vi "car proceed.vi"(0 "location in":T1, 1 "old buffer":T2, 2 "velocity in":cluster{"x":dbl, "y":dbl}, 3 "sensor reading":T3, 4 "Backward?":bool, 5 "refresh rate":i32) -> (6 "location out":T1, 8 "new buffer":T2, 9 "realdir":dbl, 10 "velocity out":cluster{"x":dbl, "y":dbl})   [LabVIEW 2020]
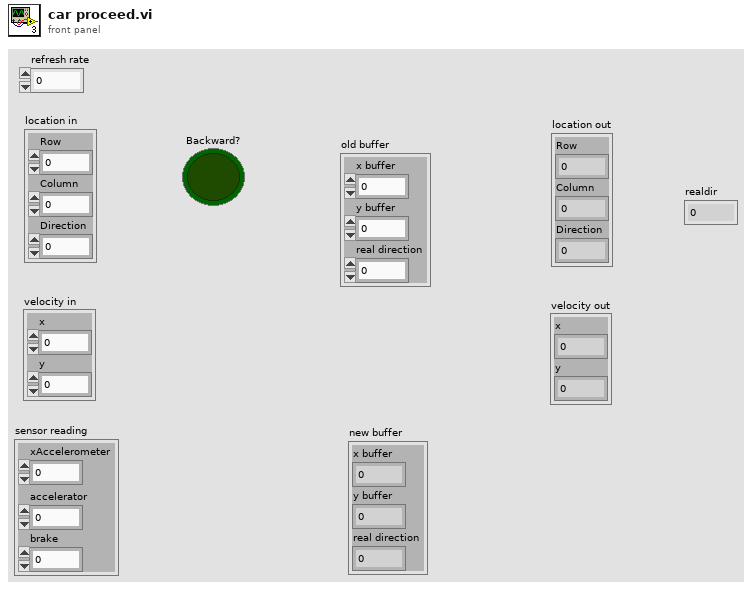
[diagram p1: front panel]
types:
  T1 = cluster{"Row":i32, "Column":i32, "Direction":i32}
  T2 = cluster{"x buffer":dbl, "y buffer":dbl, "real direction":dbl}
  T3 = cluster{"xAccelerometer":dbl, "accelerator":dbl, "brake":dbl}
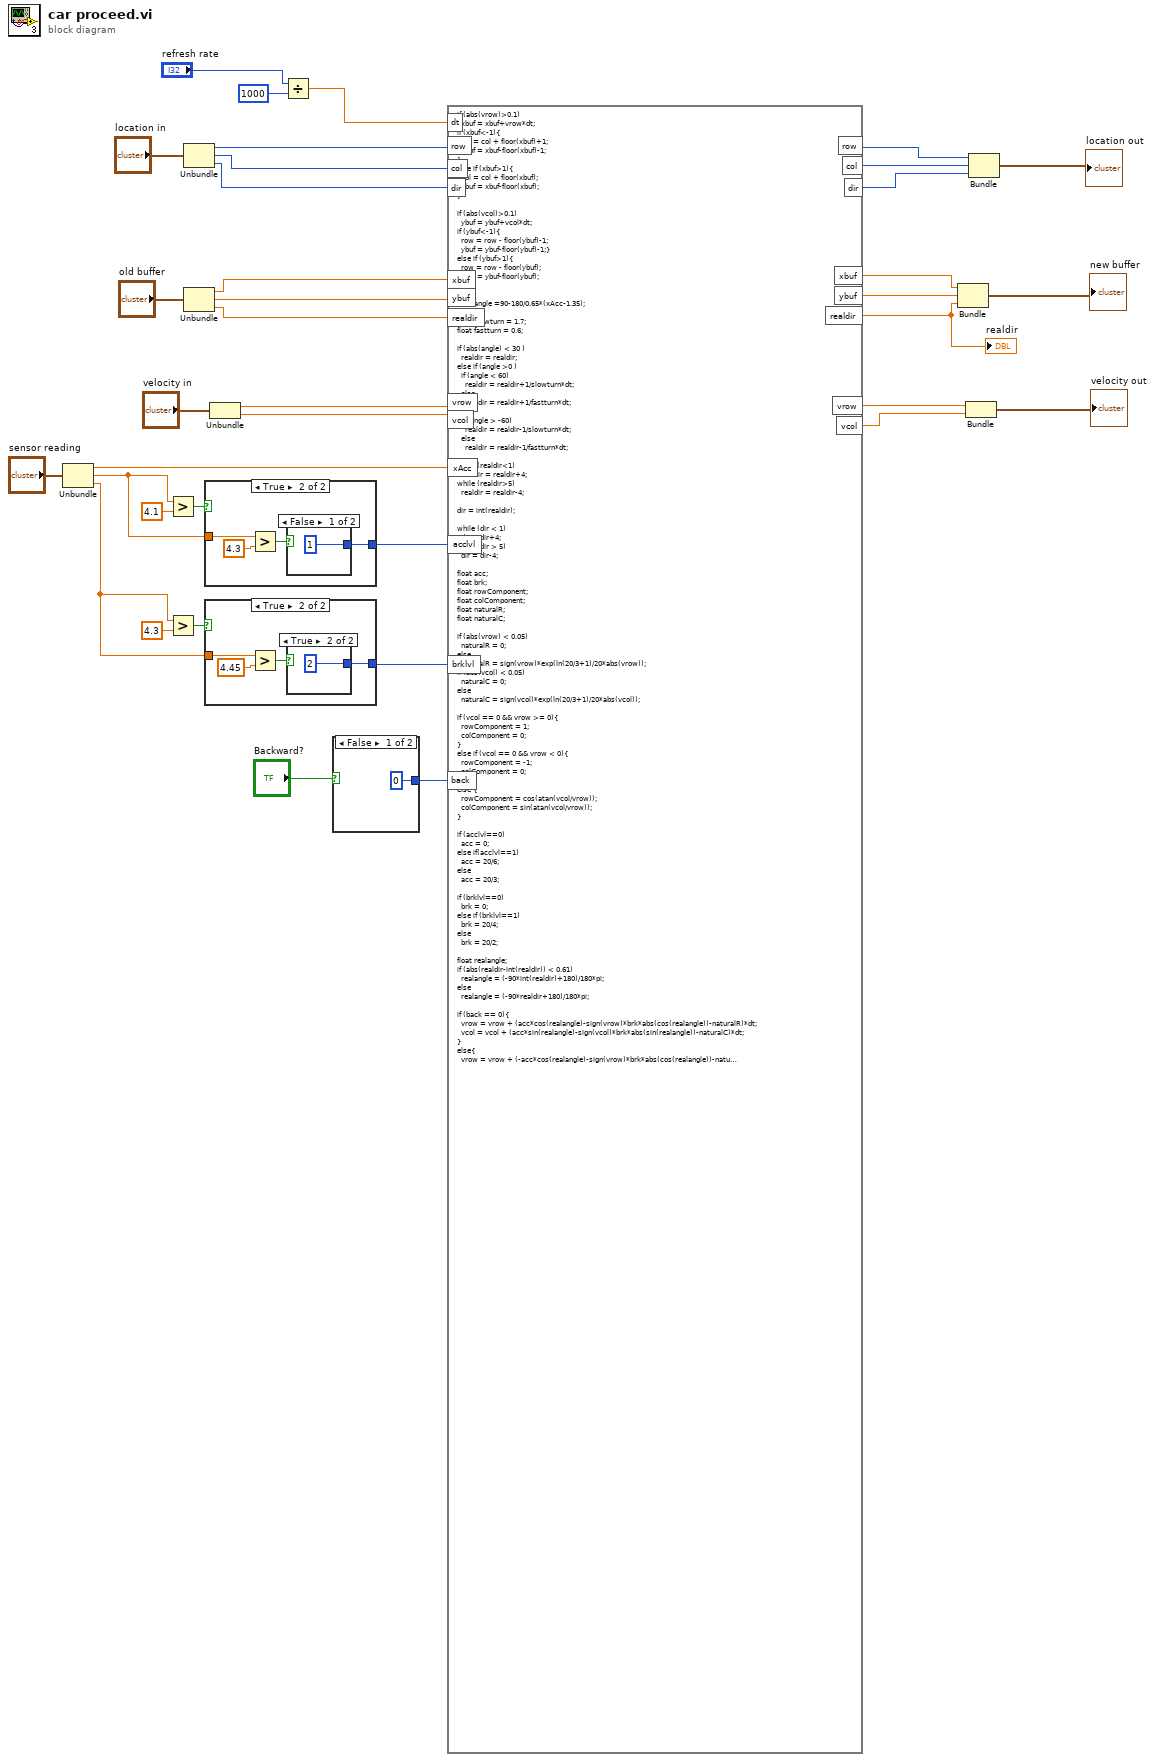
[diagram p0: block diagram]
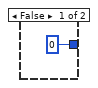
[diagram p2: hidden frame]
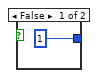
[diagram p3: hidden frame]
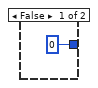
[diagram p4: hidden frame]
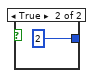
[diagram p5: hidden frame]
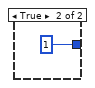
[diagram p6: hidden frame]
diagram:
  n1 = Unbundle("sensor reading") -> ("xAccelerometer"=w3:dbl, "accelerator"=w5:dbl, "brake"=w4:dbl)
  n2 = Greater?(x=w5, y=4.1) -> (0:w8:bool)
  n3 = Greater?(x=w4, y=4.3) -> (0:w7:bool)
  n4 = Unbundle("location in") -> ("Row"=w33:i32, "Column"=w32:i32, "Direction"=w31:i32)
  n5 = Unbundle("old buffer") -> ("x buffer"=w30:dbl, "y buffer"=w29:dbl, "real direction"=w28:dbl)
  n6 = case shown="True" w8 {
    tunnel: [0 w39] -> w2
    tunnel: w5 -> [_ w42]
    frame False {
    }
    frame True {
      n7 = Greater?(x=w42, y=4.3) -> (0:w40:bool)
      n8 = case shown="False" w40 {
        tunnel: [1 2] -> w39
        frame False {
        }
        frame True {
        }
      }
    }
  }
  n9 = case shown="True" w7 {
    tunnel: [0 w46] -> w1
    tunnel: w4 -> [_ w49]
    frame False {
    }
    frame True {
      n10 = Greater?(x=w49, y=4.45) -> (0:w47:bool)
      n11 = case shown="True" w47 {
        tunnel: [1 2] -> w46
        frame False {
        }
        frame True {
        }
      }
    }
  }
  n12 = Unbundle("velocity in") -> ("x"=w27:dbl, "y"=w26:dbl)
  n13 = Divide(x="refresh rate", y=1000) -> (x/y=w13:dbl)
  n14 = case shown="False" "Backward?" {
    tunnel: [0 1] -> w10
    frame False {
    }
    frame True {
    }
  }
  n15 = formula code="if (abs(vrow)>0.1)\n  xbuf = xbuf+vrow*dt;\nif (xbuf<-1){\n  col = col + floor(xbuf)+1;\n  xbuf = xbuf-floor(xbuf)-1;\n}\nelse if (xbuf>1){\n  col = col + floor(xbuf);\n  xbuf = xbuf-floor(xbuf);\n}\n\nif (abs(vcol)>0.1)\n  ybuf = ybuf+vcol*dt;\nif (ybuf<-1){\n  row = row - floor(ybuf)-1;\n  ybuf = ybuf-floor(ybuf)-1;}\nelse if (ybuf>1){\n  row = row - floor(ybuf);\n  ybuf = ybuf-floor(ybuf);\n}\n\nfloat angle =90-180/0.65*(xAcc-1.35);\n\nfloat slowturn = 1.7;\nfloat fastturn = 0.6;\n\nif (abs(angle) < 30 )\n  realdir = realdir;\nelse if (angle >0 )\n  if (angle < 60)\n    realdir = realdir+1/slowturn*dt;\n  else\n    realdir = realdir+1/fastturn*dt;\nelse\n  if (angle > -60)\n    realdir = realdir-1/slowturn*dt;\n  else\n    realdir = realdir-1/fastturn*dt;\n\nwhile (realdir<1)\n  realdir = realdir+4;\nwhile (realdir>5)\n  realdir = realdir-4;\n\ndir = int(realdir);\n\nwhile (dir < 1)\n  dir = dir+4;\nwhile (dir > 5)\n  dir = dir-4;\n\nfloat acc;\nfloat brk;\nfloat rowComponent;\nfloat colComponent;\nfloat naturalR;\nfloat naturalC;\n\nif (abs(vrow) < 0.05)\n  naturalR = 0;\nelse\n  naturalR = sign(vrow)*exp(ln(20/3+1)/20*abs(vrow));\nif (abs(vcol) < 0.05)\n  naturalC = 0;\nelse\n  naturalC = sign(vcol)*exp(ln(20/3+1)/20*abs(vcol));\n\nif (vcol == 0 && vrow >= 0){\n  rowComponent = 1;\n  colComponent = 0;\n}\nelse if (vcol == 0 && vrow < 0){\n  rowComponent = -1;\n  colComponent = 0;\n}\nelse {\n  rowComponent = cos(atan(vcol/vrow));\n  colComponent = sin(atan(vcol/vrow));\n}\n\nif (acclvl==0)\n  acc = 0;\nelse if(acclvl==1)\n  acc = 20/6;\nelse\n  acc = 20/3;\n\nif (brklvl==0)\n  brk = 0;\nelse if (brklvl==1)\n  brk = 20/4;\nelse\n  brk = 20/2;\n\nfloat realangle;\nif (abs(realdir-int(realdir)) < 0.61)\n  realangle = (-90*int(realdir)+180)/180*pi;\nelse\n  realangle = (-90*realdir+180)/180*pi;\n\nif (back == 0){\n  vrow = vrow + (acc*cos(realangle)-sign(vrow)*brk*abs(cos(realangle))-naturalR)*dt;\n  vcol = vcol + (acc*sin(realangle)-sign(vcol)*brk*abs(sin(realangle))-naturalC)*dt;\n}\nelse{\n  vrow = vrow + (-acc*cos(realangle)-sign(vrow)*brk*abs(cos(realangle))-naturalR)*dt;\n  vcol = vcol + (-acc*sin(realangle)-sign(vcol)*brk*abs(sin(realangle))-naturalC)*dt;\n}"("row"=w33, "col"=w32, "dir"=w31, "xbuf"=w30, "ybuf"=w29, "realdir"=w28, "vrow"=w27, "vcol"=w26, "xAcc"=w3, "dt"=w13, "back"=w10, "acclvl"=w2, "brklvl"=w1) -> ("row"=w25:i32, "col"=w24:i32, "dir"=w23:i32, "xbuf"=w21:dbl, "ybuf"=w20:dbl, "realdir"=w19:dbl, "vrow"=w17:dbl, "vcol"=w16:dbl)
  "realdir" <- w19
  n16 = Bundle("xbuf"=w21, "ybuf"=w20, "realdir"=w19) -> (→"new buffer":cluster{"xbuf":dbl, "ybuf":dbl, "realdir":dbl})  [unwired: 1 in]
  n17 = Bundle("vrow"=w17, "vcol"=w16) -> (→"velocity out":cluster{"vrow":dbl, "vcol":dbl})  [unwired: 1 in]
  n18 = Bundle("row"=w25, "col"=w24, "dir"=w23) -> (→"location out":cluster{"row":i32, "col":i32, "dir":i32})  [unwired: 1 in]
